vi "LEBITplc.PubSetFileLocation.vi"(0 "i ref in":refnum<vi>, 2 "i attribute in":T1, 5 "error in":errorcluster) -> (14 "i ref out":refnum<vi>, 16 "i attribute out":T1, 17 "SetFileLocationID":i32, 19 "error out":errorcluster)   [LabVIEW 2014, in "LEBITplc.lvlib"]
uses:
  LEBITplc.lvlib
  LEBITplc.i attribute.ctl
  CSlibraries/UtilityLib/UtilityLib.valueStatus.ctl
  CSlibraries-extern/DimLVEvent/LVDimInterface/LVDimInterface.lvlib
  CS_Core/CSSystem/CoreLib/CoreLib.lvlib
  CSlibraries/UtilityLib/UtilityLib.lvlib
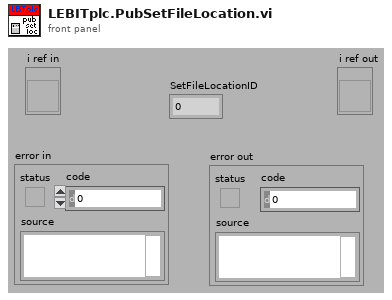
[diagram p1: front panel]
types:
  T1 = typedef "LEBITplc.lvlib/LEBITplc.i attribute.ctl" = cluster{"LLFLocation":string, "SetFileLocation":string, "nickNames":string[], "setValuePLCServiceID":i32[], "GUIServiceID":i32[], "monValuePLC":string[], "SetValueServiceID":i32[], "MonValueServiceID":i32[], "SetValue":dbl[][], "SetValueMin":dbl[], "SetValueMax":dbl[], "SetValueInfoServiceID":i32[], "GUINames":string[], "ListOfBases":string[], "Scale":dbl[], "Offset":dbl[], "setValuePLC":string[], "BaseName":string[], "ScaleServiceID":i32[], "OffsetServiceID":i32[], "AllPLCValues":string[], "CondSpecialArray":string[][], "CondSpecialIndex":i32[], "CondSpecialMonValue":dbl[], "RecentlyChanged":i32[], "SetFileLocationID":i32, "Dependent-Monitors":string[][], "LastLoadedFiles":string[], "IonGuideCalibLocation":string, "Monitor Dependent":string[], "Special":string[], "PLC?":bool[], "Start Date":string, "ListOfBasesServiceID":i32, "SETRA VISA resource":refnum<visa-resource-name>}
  T2 = typedef "UtilityLib.lvlib/UtilityLib.valueStatus.ctl" = enum16{"no info available", "stand by/off", "on", "warning", "alarm/malfunction", "not implemented", "user action required", "important information", "system default", "control default", "indicator default", "button default"}
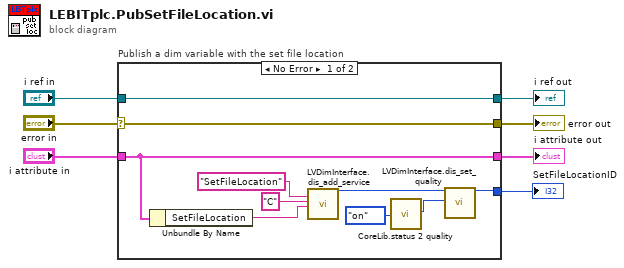
[diagram p0: block diagram]
diagram:
  n1 = case "Publish a dim variable with the set file location" shown="No Error" "error in" {
    selector: "error in" -> [w17 w19]
    tunnel: "i attribute in" -> [w15 w18]
    tunnel: [w17 w19] -> w6
    tunnel: [w16 w20] -> w5
    tunnel: "i ref in" -> [w16 w20]
    tunnel: [w15 w18] -> w2
    tunnel: [w8 _] -> w1
    frame No Error {
      n2 = Unbundle By Name(w15) -> ("SetFileLocation"=w14:string)
      n3 = call "LVDimInterface.dis_add_service.vi"("serviceName"="SetFileLocation", "typeDescriptor"="C", "data"=w14) -> ("my_serviceID"=w11:i32)  [unwired: 15 in, 1 out]
      n4 = call "CoreLib.status 2 quality.vi"("valueStatus"=UtilityLib.valueStatus."on") -> ("quality"=w13:i32)  [unwired: 18 in]
      n5 = call "LVDimInterface.dis_set_quality.vi"("my_serviceID"=w11, "quality"=w13) -> ("my_serviceID (out)"=w8:i32)  [unwired: 16 in, 1 out]
    }
    frame Error {
    }
  }
  "error out" <- w6
  "i ref out" <- w5
  "i attribute out" <- w2
  "SetFileLocationID" <- w1
